vi "Sensor.vi"(8 "error in (no error)":errorcluster) -> (0 "error out":errorcluster)   [LabVIEW 2017]
uses:
  Type Definitions/Queue FG Options.ctl
  Type Definitions/Controller Data.ctl
  Type Definitions/DB Data.ctl
  Type Definitions/DB Info.ctl
  Type Definitions/Display Data.ctl
  Type Definitions/DB Record.ctl
  Type Definitions/Display Console States.ctl
  Type Definitions/GUI Data.ctl
  Type Definitions/Controller States.ctl
  Type Definitions/Sensor UI Data.ctl
  Type Definitions/Controller Message.ctl
panel:
  in  "Funds dispensed":bool
  in  "Deposit received":bool
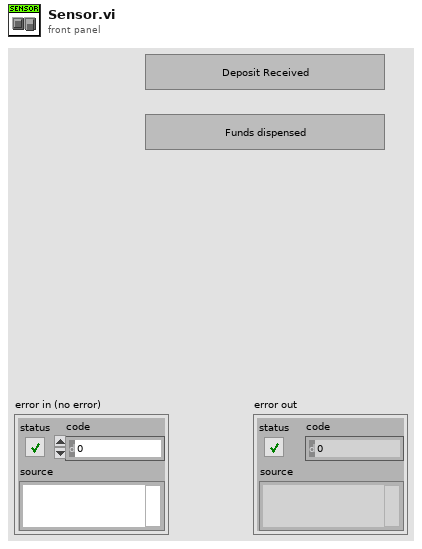
[diagram p1: front panel]
types:
  T1 = typedef "Queue FG Options.ctl" = enum16{"Set", "Get", "Read", "Write", "Destroy"}
  T2 = typedef "Controller States.ctl" = enum16{"Timeout", "Initial", "Login", "Idle", "Balance Inquiry", "Deposit", "Withdrawal", "Fast Cash", "Terminate", "Wait on Exit", "Shutdown", "Error Handler"}
  T3 = typedef "Controller Message.ctl" = cluster{"Message Info":T2, "Message Data":variant}
  T4 = typedef "Controller Data.ctl" = cluster{"Time":dbl, "DB Data in":T5, "Display Data":T7, "GUI Data ":T10, "Sensor UI":T11, "Controller States":T2}
  T5 = typedef "DB Data.ctl" = cluster{"Account":i32, "First Name":string, "Last Name":string, "Balance":fxp<+/-,64,35>, "DB Info":T6}
  T6 = typedef "DB Info.ctl" = enum16{"Empty", "Verify", "Login Accepted", "Invalid Login", "Deposit Complete", "Withdrawal Complete", "Withdrawal Failed", "Terminate"}
  T7 = typedef "Display Data.ctl" = cluster{"Message Text":string, "DB Record":T8, "Card Read":bool, "Display Console States":T9}
  T8 = typedef "DB Record.ctl" = cluster{"Account":i32, "First Name":string, "Last Name":string, "Balance":fxp<+/-,64,35>}
  T9 = typedef "Display Console States.ctl" = enum16{"Timeout", "Initial", "Login", "Invalid Login", "Idle", "Balance Inquiry", "Deposit", "Withdrawal", "Fast Cash", "Withdrawal Failed", "Withdrawal Complete", "Terminate", "Shutdown"}
  T10 = typedef "GUI Data.ctl" = cluster{"Card Reader":enum8{"Enabled", "Disabled", "Disabled and Grayed Out"}, "Keypad":enum8{"Enabled", "Disabled", "Disabled and Grayed Out"}, "Balance Inquiry":enum8{"Enabled", "Disabled", "Disabled and Grayed Out"}, "Deposit":enum8{"Enabled", "Disabled", "Disabled and Grayed Out"}, "Withdrawal":enum8{"Enabled", "Disabled", "Disabled and Grayed Out"}, "Fast Cash":enum8{"Enabled", "Disabled", "Disabled and Grayed Out"}, "New Transaction":enum8{"Enabled", "Disabled", "Disabled and Grayed Out"}, "Terminate Session":enum8{"Enabled", "Disabled", "Disabled and Grayed Out"}, "Pinpad Value":string, "Timeout":i32, "Controller States":T2}
  T11 = typedef "Sensor UI Data.ctl" = cluster{"Funds dispensed":enum16{"Enabled", "Disabled", "Disabled and Grayed Out"}, "Deposit received":enum16{"Enabled", "Disabled", "Disabled and Grayed Out"}, "Timeout":dbl}
  T12 = typedef "Sensor States.ctl" = enum16{"Initial", "Idle", "Shutdown"}
  T13 = enum16{"Enabled", "Disabled", "Disabled and Grayed Out"}
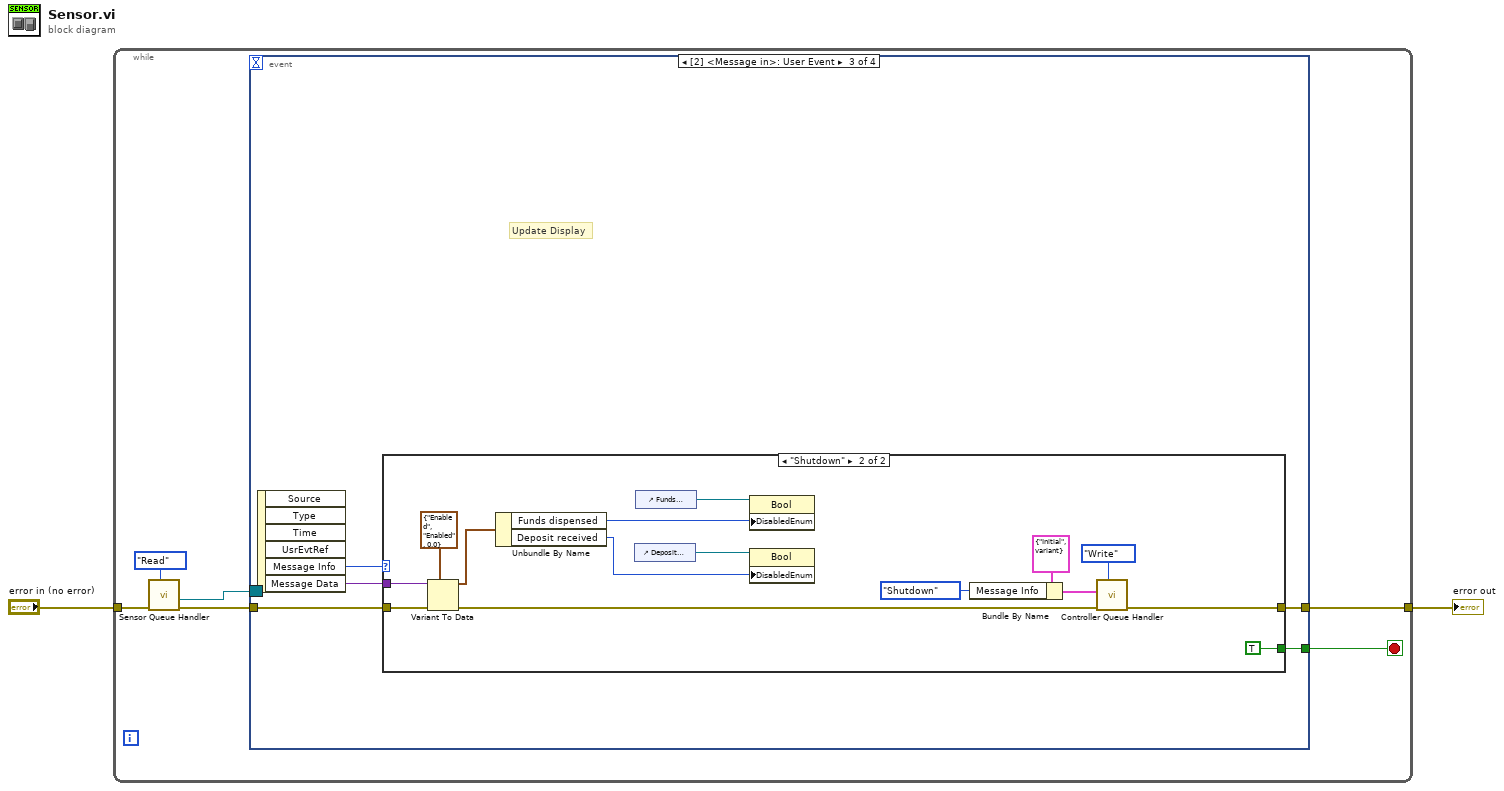
[diagram p0: block diagram]
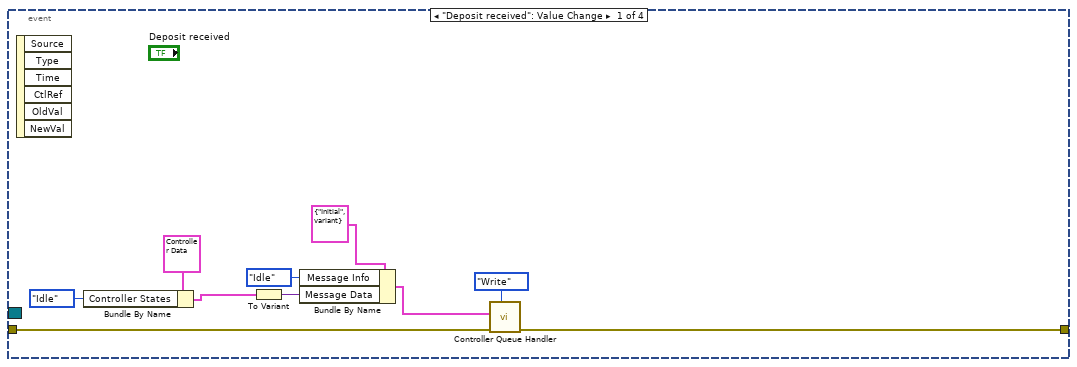
[diagram p2: hidden frame]
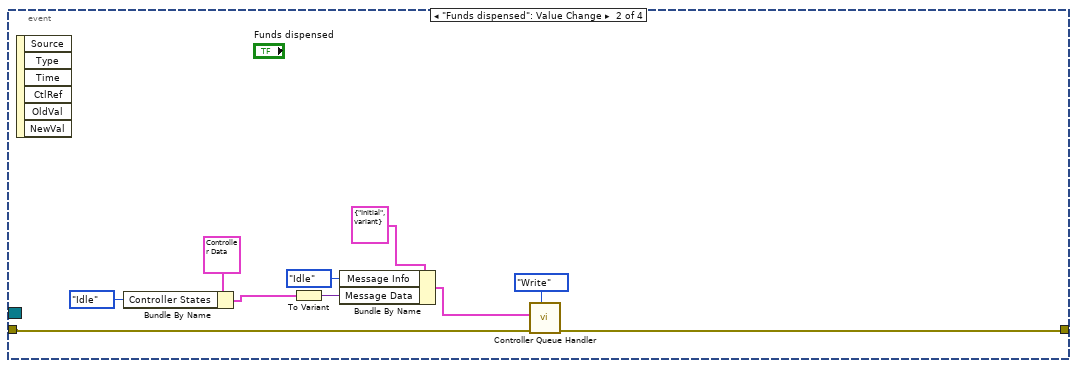
[diagram p3: hidden frame]
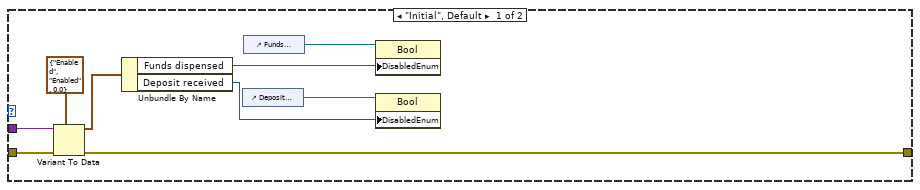
[diagram p4: hidden frame]
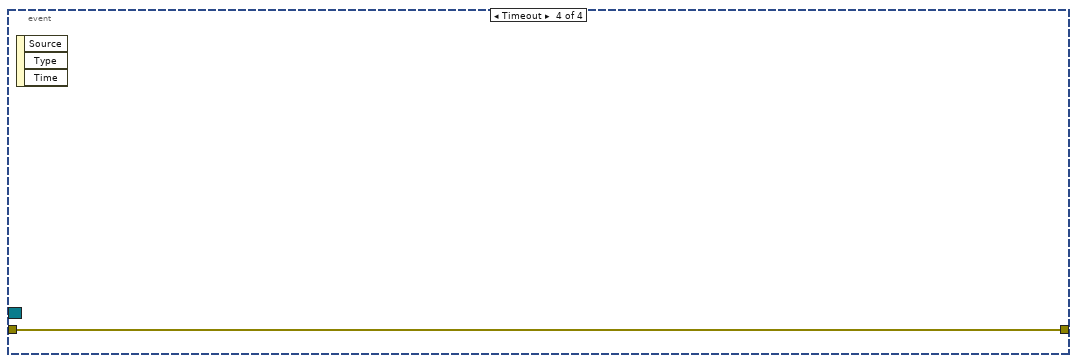
[diagram p5: hidden frame]
diagram:
  n1 = while {
    tunnel: "error in (no error)" -> [w7]
    tunnel: [w5] -> w1
    stop <- w3 stop-if-true
    n2 = call "Sensor Queue Handler.vi"("Action"=Queue_FG_Options."Read", "error in (no error)"=w7) -> ("error out"=w6:errorcluster, "Event Registration Refnum"=w4:refnum<event-registration>)  [unwired: 6 in, 2 out]
    n3 = event shown="[2] <Message in>: User Event" {
      selector: w4 -> [_ _ _ _]
      dyn-events: _ -> [_ _ _ _]
      timeout: _ -> [_ _ _ _]
      tunnel: w6 -> [w18 w20 w33 w58]
      tunnel: [w17 w19 w32 w58] -> w5
      tunnel: [_ _ w31 _] -> w3
      event "Deposit received": Value Change {
        n4 = event-data() -> ()  [unwired: 1 in, 6 out]
        n5 = Bundle By Name(cluster=T4 {"Time"=0.0, "DB Data in"={"Account"=0, "First Name"="", "Last Name"="", "Balance"=0.0, "DB Info"=enum."Login Accepted"}, "Display Data"={"Message Text"="", "DB Record"={"Account"=0, "First Name"="", "Last Name"="", "Balance"=0.0}, "Card Read"=FALSE, "Display Console States"=enum."Timeout"}, "GUI Data "={"Card Reader"=enum."Enabled", "Keypad"=enum."Enabled", "Balance Inquiry"=enum."Enabled", "Deposit"=enum."Enabled", "Withdrawal"=enum."Enabled", "Fast Cash"=enum."Enabled", "New Transaction"=enum."Enabled", "Terminate Session"=enum."Enabled", "Pinpad Value"="", "Timeout"=0, "Controller States"=enum."Initial"}, "Sensor UI"={"Funds dispensed"=enum."Enabled", "Deposit received"=enum."Enabled", "Timeout"=0.0}, "Controller States"=enum."Timeout"} ("Controller Data"), "Controller States"=Controller_States."Idle") -> (w11:T4)
        n6 = To Variant(anything=w11) -> (Variant=w10:variant)
        n7 = Bundle By Name(cluster=T3 {"Message Info"=enum."Initial", "Message Data"=variant} ("Message"), "Message Info"=Controller_States."Idle", "Message Data"=w10) -> (w9:T3)
        n8 = call "Controller Queue Handler.vi"("Action"=Queue_FG_Options."Write", "error in (no error)"=w18, "Message in"=w9) -> ("error out"=w17:errorcluster)  [unwired: 6 in, 2 out]
      }
      event "Funds dispensed": Value Change {
        n9 = event-data() -> ()  [unwired: 1 in, 6 out]
        n10 = Bundle By Name(cluster=T4 {"Time"=0.0, "DB Data in"={"Account"=0, "First Name"="", "Last Name"="", "Balance"=0.0, "DB Info"=enum."Login Accepted"}, "Display Data"={"Message Text"="", "DB Record"={"Account"=0, "First Name"="", "Last Name"="", "Balance"=0.0}, "Card Read"=FALSE, "Display Console States"=enum."Timeout"}, "GUI Data "={"Card Reader"=enum."Enabled", "Keypad"=enum."Enabled", "Balance Inquiry"=enum."Enabled", "Deposit"=enum."Enabled", "Withdrawal"=enum."Enabled", "Fast Cash"=enum."Enabled", "New Transaction"=enum."Enabled", "Terminate Session"=enum."Enabled", "Pinpad Value"="", "Timeout"=0, "Controller States"=enum."Initial"}, "Sensor UI"={"Funds dispensed"=enum."Enabled", "Deposit received"=enum."Enabled", "Timeout"=0.0}, "Controller States"=enum."Timeout"} ("Controller Data"), "Controller States"=Controller_States."Idle") -> (w23:T4)
        n11 = To Variant(anything=w23) -> (Variant=w22:variant)
        n12 = Bundle By Name(cluster=T3 {"Message Info"=enum."Initial", "Message Data"=variant} ("Message"), "Message Info"=Controller_States."Idle", "Message Data"=w22) -> (w21:T3)
        n13 = call "Controller Queue Handler.vi"("Action"=Queue_FG_Options."Write", "error in (no error)"=w20, "Message in"=w21) -> ("error out"=w19:errorcluster)  [unwired: 6 in, 2 out]
      }
      event User Event {
        # "Update Display"
        n14 = event-data() -> ("Message Info"=w29:T12, "Message Data"=w30:variant)  [unwired: 1 in, 4 out]
        n15 = case shown="\"Shutdown\"" w29 {
          tunnel: w33 -> [w42 w57]
          tunnel: [w41 w47] -> w32
          tunnel: w30 -> [w40 w55]
          tunnel: [_ TRUE] -> w31
          frame "Initial", Default {
            n16 = Variant To Data(error in=w42, type=T11 {"Funds dispensed"=enum."Enabled", "Deposit received"=enum."Enabled", "Timeout"=0.0} ("Sensor UI"), Variant=w40) -> (data=w38:T11, error out=w41:errorcluster)
            n17 = Unbundle By Name(w38) -> ("Funds dispensed"=w37:T13, "Deposit received"=w36:T13)
            n18 = control-ref of="Deposit received"() -> (w34:refnum<vi>)
            n19 = control-ref of="Funds dispensed"() -> (w35:refnum<vi>)
            n20 = property class="Bool"(reference=w35, "DisabledEnum"=w37) -> ()  [unwired: 1 in, 2 out]
            n21 = property class="Bool"(reference=w34, "DisabledEnum"=w36) -> ()  [unwired: 1 in, 2 out]
          }
          frame "Shutdown" {
            n22 = Variant To Data(error in=w57, type=T11 {"Funds dispensed"=enum."Enabled", "Deposit received"=enum."Enabled", "Timeout"=0.0} ("Sensor UI"), Variant=w55) -> (data=w53:T11, error out=w56:errorcluster)
            n23 = Unbundle By Name(w53) -> ("Funds dispensed"=w52:T13, "Deposit received"=w51:T13)
            n24 = control-ref of="Deposit received"() -> (w48:refnum<vi>)
            n25 = control-ref of="Funds dispensed"() -> (w49:refnum<vi>)
            n26 = property class="Bool"(reference=w49, "DisabledEnum"=w52) -> ()  [unwired: 1 in, 2 out]
            n27 = property class="Bool"(reference=w48, "DisabledEnum"=w51) -> ()  [unwired: 1 in, 2 out]
            n28 = Bundle By Name(cluster=T3 {"Message Info"=enum."Initial", "Message Data"=variant} ("Message"), "Message Info"=Controller_States."Shutdown") -> (w44:T3)
            n29 = call "Controller Queue Handler.vi"("Action"=Queue_FG_Options."Write", "error in (no error)"=w56, "Message in"=w44) -> ("error out"=w47:errorcluster)  [unwired: 6 in, 2 out]
          }
        }
      }
      event Timeout {
        n30 = event-data() -> ()  [unwired: 1 in, 3 out]
      }
    }
  }
  "error out" <- w1
